vi "DrawChessboardSemiCircleSquare.vi"(0 "Bounds":T2, 1 "Skip":bool, 4 "picture in":picture, 5 "Semi Circle Square Type":T1) -> (7 "picture out":picture)   [LabVIEW 2020, in "ar.lvlib"]
uses:
  ar.lvlib
  Chessboard Semi Circle Square Type.ctl
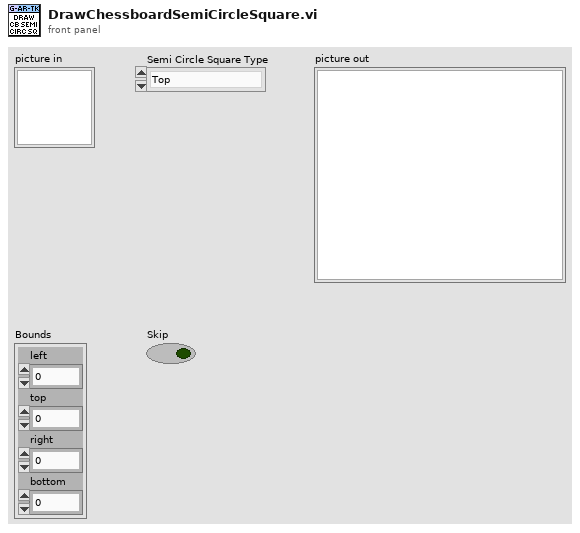
[diagram p1: front panel]
types:
  T1 = typedef "ar.lvlib/Chessboard Semi Circle Square Type.ctl" = enum16{"Top", "Left", "Right", "Bottom"}
  T2 = cluster{"left":i16, "top":i16, "right":i16, "bottom":i16}
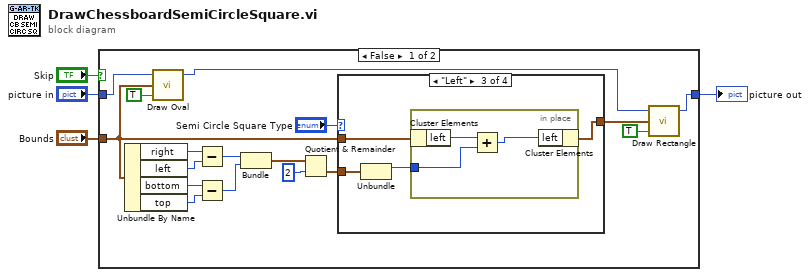
[diagram p0: block diagram]
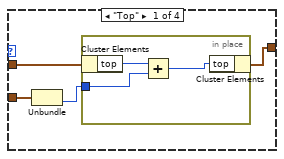
[diagram p2: hidden frame]
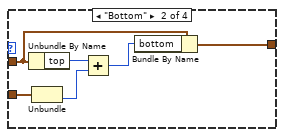
[diagram p3: hidden frame]
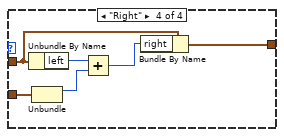
[diagram p4: hidden frame]
diagram:
  n1 = case shown="False" "Skip" {
    tunnel: [w20 w48] -> w4
    tunnel: "picture in" -> [w17 w48]
    tunnel: "Bounds" -> [w7 _]
    frame False {
      n2 = Unbundle By Name(w7) -> ("right"=w16:i16, "left"=w15:i16, "bottom"=w14:i16, "top"=w13:i16)
      n3 = call <vilib>:"Draw Oval.vi"("picture"=w17, "rect"=w7, "fill?(F)"=TRUE) -> ("new picture"=w19:picture)  [unwired: 6 in]
      n4 = Subtract(x=w16, y=w15) -> (x-y=w12:i16)
      n5 = Subtract(x=w14, y=w13) -> (x-y=w11:i16)
      n6 = Bundle(w12, w11) -> (w10:cluster{i16, i16})  [unwired: 1 in]
      n7 = Quotient & Remainder(x=w10, y=i16 2) -> (floor(x/y)=w6:cluster{i16, i16})  [unwired: 1 out]
      n8 = case shown="\"Left\"" "Semi Circle Square Type" {
        tunnel: w7 -> [w23 w33 w36 w46]
        tunnel: w6 -> [w25 w32 w38 w45]
        tunnel: [w22 w34 w35 w47] -> w5
        frame "Top" {
          n9 = Unbundle(w25) -> (w24:i16)  [unwired: 1 out]
          n10 = in-place {
            in-place-border: w24 -> [w28]
            n11 = in-place-cluster #1(w23) -> ("top"=w26:i16)
            n12 = Add(x=w26, y=w28) -> (x+y=w27:i16)
            n13 = in-place-cluster #1("top"=w27) -> (w22:T2)
          }
        }
        frame "Bottom" {
          n14 = Unbundle By Name(w33) -> ("top"=w31:i16)
          n15 = Unbundle(w32) -> (w30:i16)  [unwired: 1 out]
          n16 = Add(x=w31, y=w30) -> (x+y=w29:i16)
          n17 = Bundle By Name(cluster=w33, "bottom"=w29) -> (w34:T2)
        }
        frame "Left" {
          n18 = Unbundle(w38) -> (w37:i16)  [unwired: 1 out]
          n19 = in-place {
            in-place-border: w37 -> [w41]
            n20 = in-place-cluster #2(w36) -> ("left"=w40:i16)
            n21 = Add(x=w40, y=w41) -> (x+y=w39:i16)
            n22 = in-place-cluster #2("left"=w39) -> (w35:T2)
          }
        }
        frame "Right" {
          n23 = Unbundle By Name(w46) -> ("left"=w44:i16)
          n24 = Unbundle(w45) -> (w42:i16)  [unwired: 1 out]
          n25 = Add(x=w44, y=w42) -> (x+y=w43:i16)
          n26 = Bundle By Name(cluster=w46, "right"=w43) -> (w47:T2)
        }
      }
      n27 = call <vilib>:"Draw Rectangle.vi"("picture"=w19, "rect"=w5, "fill?(F)"=TRUE) -> ("new picture"=w20:picture)  [unwired: 6 in]
    }
    frame True {
    }
  }
  "picture out" <- w4
